vi "read version.vi"(11 "Builder in":refnum<class "Builder.lvclass">) -> (2 "version":T1)   [LabVIEW 2024, in "Builder.lvclass"]
uses:
  Builder.lvclass
  Builder.lvclass/Builder.ctl
  <vilib>/AppBuilder/AB_API/common/AB_API Version Number.ctl
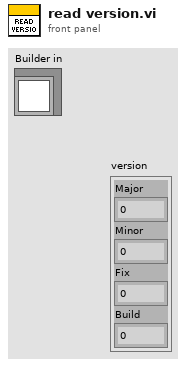
[diagram p1: front panel]
types:
  T1 = typedef "AB_API Version Number.ctl" = cluster{"Major":u16, "Minor":u16, "Fix":u16, "Build":u16}
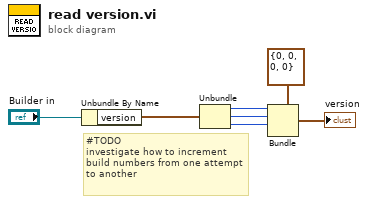
[diagram p0: block diagram]
diagram:
  # "#TODO\ninvestigate how to increment build numbers from one attempt to another"
  n1 = Unbundle By Name("Builder in") -> ("version"=w3:cluster{"major":u16, "minor":u16, "bugfix":u16})
  n2 = Unbundle(w3) -> ("major"=w6:u16, "minor"=w5:u16, "bugfix"=w4:u16)
  n3 = Bundle(cluster=T1 {"Major"=0, "Minor"=0, "Fix"=0, "Build"=0} ("version"), "Major"=w6, "Minor"=w5, "Fix"=w4) -> (→"version":T1)  [unwired: 1 in]
